vi "Write Name.vi"(8 "error in":errorcluster, 10 "name":string, 11 "module in":refnum<class "Module.lvclass">) -> (0 "error out":errorcluster, 3 "module out":refnum<class "Module.lvclass">)   [LabVIEW 2019, in "Scan Engine Scripting.lvlib" / "Module.lvclass"]
uses:
  Module.lvclass
  Module.lvclass/Module.ctl
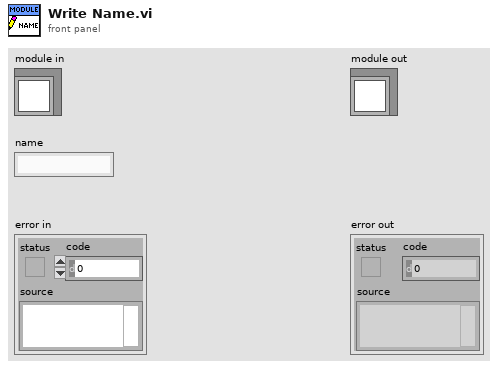
[diagram p1: front panel]
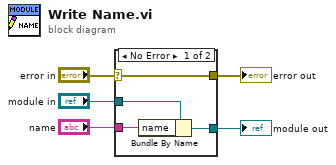
[diagram p0: block diagram]
diagram:
  n1 = case shown="No Error" "error in" {
    selector: "error in" -> [w9 w10]
    tunnel: [w9 w10] -> w4
    tunnel: [w7 w11] -> w2
    tunnel: "module in" -> [w8 w11]
    tunnel: "name" -> [w6 _]
    frame No Error {
      n2 = Bundle By Name(cluster=w8, "name"=w6) -> (w7:refnum<class "Module.lvclass">)
    }
    frame Error {
    }
  }
  "error out" <- w4
  "module out" <- w2
